vi "SYST_UPR_PNA.vi"(0 "VISA IN":refnum<visa-resource-name>, 5 "error in":errorcluster) -> (14 "VISA Out":refnum<visa-resource-name>, 19 "error out":errorcluster)   [LabVIEW 2018, in "PNA-X.lvlib"]
doc: "SYSTem:UPReset will cause the PNA to assume this instrument state. \nRegardless of the state of the User Preset Enable checkbox, the SYST:PRESet command will always \npreset the PNA to the factory preset settings, and SYST:UPReset will always perform a User Preset. \nLearn more about User Preset. \nExamples SYST:UPR:SAVE \nsystem:upreset:save:state \nQuery Syntax Not Applicable \nDefault Not Applicable"
uses:
  PNA-X.lvlib
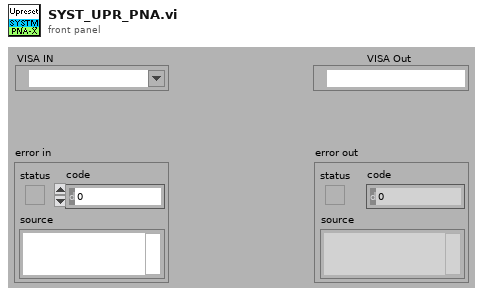
[diagram p1: front panel]
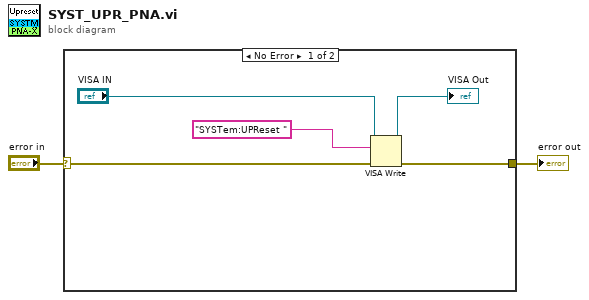
[diagram p0: block diagram]
diagram:
  n1 = case shown="No Error" "error in" {
    selector: "error in" -> [w4 w8]
    tunnel: [w6 w8] -> w1
    frame No Error {
      n2 = VISA Write(VISA resource name="VISA IN", write buffer="SYSTem:UPReset " ("Cmdline"), error in (no error)=w4) -> (VISA resource name out=→"VISA Out":refnum<visa-resource-name>, error out=w6:errorcluster)  [unwired: 1 out]
    }
    frame Error {
    }
  }
  "error out" <- w1
